vi "Finish.vi"(4 "error in (no error)":errorcluster) -> (0 "error out":errorcluster)   [LabVIEW 2016]
doc: "This VI is called just before exiting. It is expected to close I/O refnum, save collected data, etc."
uses:
  <vilib>/Rock Robotics/WPI/Utilities/WPI_GetSetVariantRefNum.vi
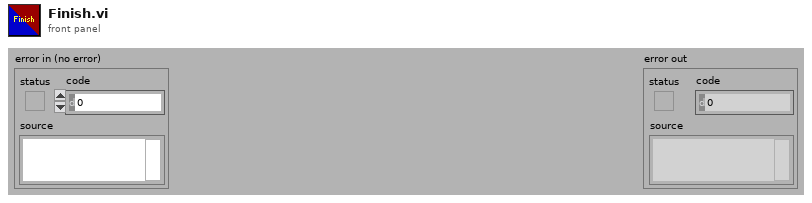
[diagram p1: front panel]
types:
  T1 = typedef "WPI_SolenoidDevRef.ctl" = cluster{"DevStatus":errorcluster, "Pneumatics Control Module":u8, "Forward Solenoid Channel":T2, "Reverse Solenoid Channel":T2}
  T2 = typedef "WPI_SolenoidChannel.ctl" = enum8{"Solenoid 0", "Solenoid 1", "Solenoid 2", "Solenoid 3", "Solenoid 4", "Solenoid 5", "Solenoid 6", "Solenoid 7", "Invalid"}
  T3 = typedef "WPI_JoystickDevRef.ctl" = cluster{"Device":T4}
  T4 = typedef "WPI_JoystickDeviceEnum.ctl" = enum16{"USB 0", "USB 1", "USB 2", "USB 3", "USB 4", "USB 5"}
  T5 = typedef "WPI_GyroDevRef.ctl" = cluster{"DevStatus":errorcluster, "Analog Channel":T6, "Offset":dbl, "Gain (VoltsPerDegree/Second)":dbl, "Gyro Type":enum16{"Analog", "XRS450"}, "Handle":i32, "SPI Bus":T7, "Device Found":bool, "Sample Rate":dbl, "Calibrate On Open":bool}
  T6 = typedef "FPGA_AIChannel.ctl" = enum8{"AI 0", "AI 1", "AI 2", "AI 3", "AI MXP 0", "AI MXP 1", "AI MXP 2", "AI MXP 3", "Invalid"}
  T7 = typedef "spi_bus.ctl" = enum16{"SPI On-Board, CS0", "SPI On-Board, CS1", "SPI On-Board, CS2", "SPI On-Board, CS3", "SPI MXP", "Invalid"}
  T8 = typedef "WPI_AccelerometerDevRef.ctl" = cluster{"DevStatus":errorcluster, "Scaling":T9, "Analog Channels":T10, "I2C Bus":T11, "SPI Bus":T7, "Accel Range":T12, "ADXL Axes":T13, "Handle":i32, "Device Address":u8, "Accel Type":enum16{"Analog", "ADXL345 I2C", "ADXL345 SPI", "Internal", "ADXL362 SPI"}}
  T9 = typedef "WPI_AccelerometerScaling.ctl" = cluster{"Gain (VoltsPerG)":dbl, "Center Voltage":dbl}
  T10 = typedef "WPI_AccelerometerAnalogChannels.ctl" = cluster{"X-Axis":T6, "Y-Axis":T6, "Z-Axis":T6}
  T11 = typedef "i2c_bus.ctl" = enum16{"I2C On-Board", "I2C MXP", "Invalid"}
  T12 = typedef "ADXL345 Range.ctl" = u8
  T13 = typedef "WPI_AccelerometerADXL345 Axes.ctl" = cluster{"X-Axis":bool, "Y-Axis":bool, "Z-Axis":bool}
  T14 = typedef "WPI_MotorControlDeviceRef.ctl" = cluster{"DeviceStatus":errorcluster, "Type":T15, "PWM":cluster{"PWM Channel":T16, "DeadBand":T17}, "CAN":cluster{"Device Number":u8, "SetOutput VI Ref":variant, "GetOutput VI Ref":variant, "Enable VI Ref":variant, "Disable VI Ref":variant, "Data":variant}, "Invert":bool}
  T15 = typedef "WPI_MotorControlType.ctl" = enum16{"PWM", "CAN"}
  T16 = typedef "FPGA_DIOPWMChannel.ctl" = enum8{"PWM 0", "PWM 1", "PWM 2", "PWM 3", "PWM 4", "PWM 5", "PWM 6", "PWM 7", "PWM 8", "PWM 9", "PWM MXP 0", "PWM MXP 1", "PWM MXP 2", "PWM MXP 3", "PWM MXP 4", "PWM MXP 5", "PWM MXP 6", "PWM MXP 7", "PWM MXP 8", "PWM MXP 9", "Invalid"}
  T17 = typedef "WPI_PWMDeadband.ctl" = cluster{"Name":string, "maxPositivePwm":i32, "minPositivePwm":i32, "centerPwm":i32, "maxNegativePwm":i32, "minNegativePwm":i32, "angularRange":u16}
  T18 = typedef "WPI_CompressorDevRef.ctl" = cluster{"DevStatus":errorcluster, "Pneumatics Control Module":u8}
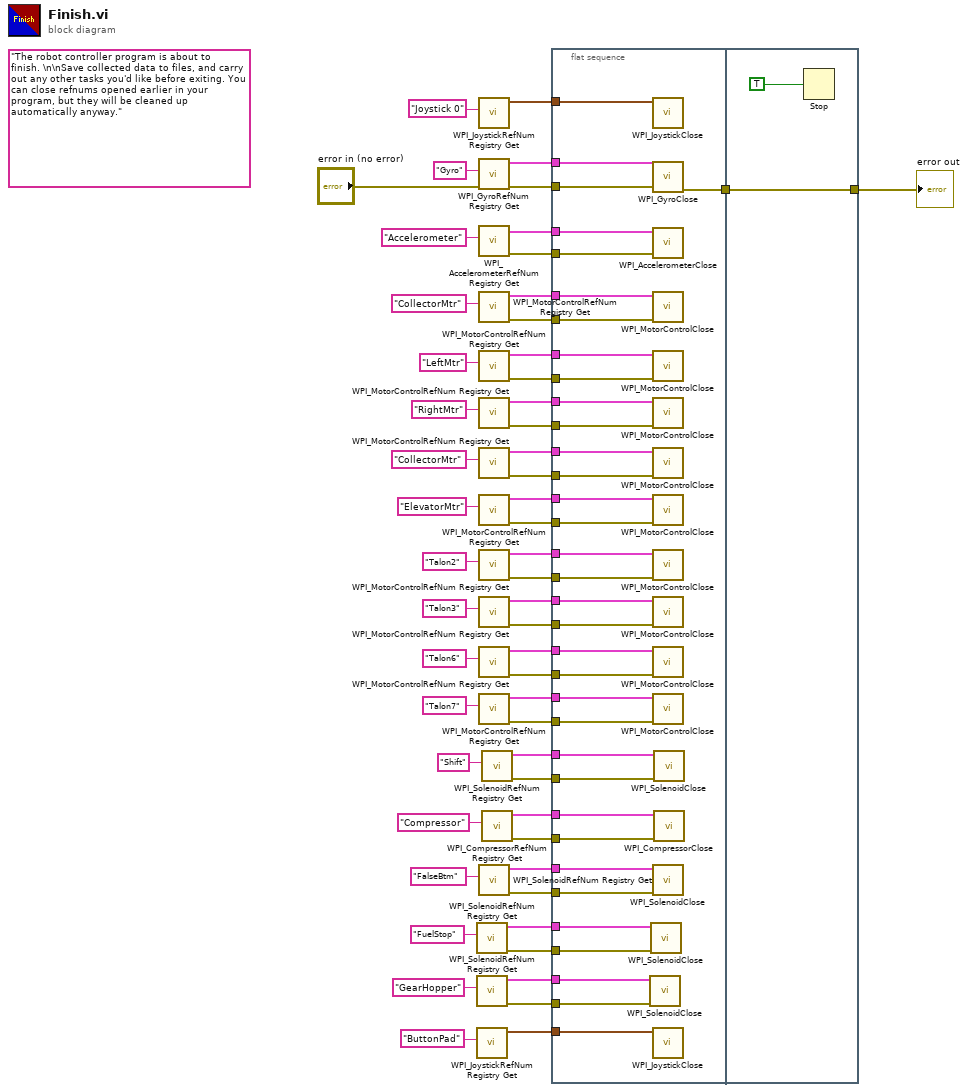
[diagram p0: block diagram]
diagram:
  (unwired) "The robot controller program is about to finish. \n\nSave collected data to files, and carry out any other tasks you'd like before exiting. You can close refnums opened earlier in your program, but they will be cleaned up automatically anyway."
  n1 = call <vilib>:"WPI_SolenoidRefNum Registry Get.vi"("refnum name"="FuelStop") -> ("error out"=w7:errorcluster, "SolenoidDevRef"=w8:T1)  [unwired: 9 in]
  n2 = call <vilib>:"WPI_SolenoidRefNum Registry Get.vi"("refnum name"="GearHopper") -> ("error out"=w9:errorcluster, "SolenoidDevRef"=w10:T1)  [unwired: 9 in]
  n3 = call <vilib>:"WPI_JoystickRefNum Registry Get.vi"("refnum name"="ButtonPad") -> ("JoystickDevRef"=w1:T3)  [unwired: 1 in, 9 out]
  n4 = call <vilib>:"WPI_JoystickRefNum Registry Get.vi"("refnum name"="Joystick 0") -> ("JoystickDevRef"=w54:T3)  [unwired: 1 in, 9 out]
  n5 = call <vilib>:"WPI_GyroRefNum Registry Get.vi"("error in (no error)"="error in (no error)", "refnum name"="Gyro") -> ("error out"=w3:errorcluster, "GyroDevRef"=w53:T5)  [unwired: 8 in]
  n6 = call <vilib>:"WPI_AccelerometerRefNum Registry Get.vi"("refnum name"="Accelerometer") -> ("error out"=w50:errorcluster, "AccelerometerDevRef"=w51:T8)  [unwired: 9 in]
  n7 = call <vilib>:"WPI_MotorControlRefNum Registry Get.vi"("refnum name"="CollectorMtr") -> ("error out"=w48:errorcluster, "MotorControlDevRef"=w47:T14)  [unwired: 9 in]
  n8 = call <vilib>:"WPI_MotorControlRefNum Registry Get.vi"("refnum name"="LeftMtr") -> ("error out"=w44:errorcluster, "MotorControlDevRef"=w43:T14)  [unwired: 9 in]
  n9 = call <vilib>:"WPI_MotorControlRefNum Registry Get.vi"("refnum name"="RightMtr") -> ("error out"=w41:errorcluster, "MotorControlDevRef"=w42:T14)  [unwired: 9 in]
  n10 = call <vilib>:"WPI_MotorControlRefNum Registry Get.vi"("refnum name"="CollectorMtr") -> ("error out"=w35:errorcluster, "MotorControlDevRef"=w36:T14)  [unwired: 9 in]
  n11 = call <vilib>:"WPI_MotorControlRefNum Registry Get.vi"("refnum name"="ElevatorMtr") -> ("error out"=w38:errorcluster, "MotorControlDevRef"=w37:T14)  [unwired: 9 in]
  n12 = call <vilib>:"WPI_MotorControlRefNum Registry Get.vi"("refnum name"="Talon2") -> ("error out"=w26:errorcluster, "MotorControlDevRef"=w27:T14)  [unwired: 9 in]
  n13 = call <vilib>:"WPI_MotorControlRefNum Registry Get.vi"("refnum name"="Talon3") -> ("error out"=w29:errorcluster, "MotorControlDevRef"=w28:T14)  [unwired: 9 in]
  n14 = call <vilib>:"WPI_MotorControlRefNum Registry Get.vi"("refnum name"="Talon6") -> ("error out"=w33:errorcluster, "MotorControlDevRef"=w32:T14)  [unwired: 9 in]
  n15 = call <vilib>:"WPI_MotorControlRefNum Registry Get.vi"("refnum name"="Talon7") -> ("error out"=w30:errorcluster, "MotorControlDevRef"=w31:T14)  [unwired: 9 in]
  n16 = call <vilib>:"WPI_SolenoidRefNum Registry Get.vi"("refnum name"="FalseBtm") -> ("error out"=w20:errorcluster, "SolenoidDevRef"=w21:T1)  [unwired: 9 in]
  n17 = call <vilib>:"WPI_SolenoidRefNum Registry Get.vi"("refnum name"="Shift") -> ("error out"=w15:errorcluster, "SolenoidDevRef"=w16:T1)  [unwired: 9 in]
  n18 = call <vilib>:"WPI_CompressorRefNum Registry Get.vi"("refnum name"="Compressor") -> ("error out"=w13:errorcluster, "CompressorDevRef"=w14:T18)  [unwired: 9 in]
  n19 = flat-sequence {
    tunnel: w54 -> [w90]
    tunnel: w53 -> [w89]
    tunnel: w51 -> [w88]
    tunnel: w50 -> [w87]
    tunnel: w48 -> [w86]
    tunnel: w47 -> [w85]
    tunnel: w44 -> [w84]
    tunnel: w43 -> [w83]
    tunnel: w41 -> [w81]
    tunnel: w42 -> [w82]
    tunnel: w35 -> [w77]
    tunnel: w36 -> [w78]
    tunnel: w38 -> [w80]
    tunnel: w37 -> [w79]
    tunnel: w26 -> [w69]
    tunnel: w27 -> [w70]
    tunnel: w29 -> [w72]
    tunnel: w28 -> [w71]
    tunnel: w33 -> [w76]
    tunnel: w32 -> [w75]
    tunnel: w30 -> [w73]
    tunnel: w31 -> [w74]
    tunnel: w20 -> [w67]
    tunnel: w21 -> [w68]
    tunnel: w16 -> [w66]
    tunnel: w15 -> [w65]
    tunnel: w14 -> [w64]
    tunnel: w13 -> [w63]
    tunnel: w10 -> [w62]
    tunnel: w9 -> [w61]
    tunnel: w8 -> [w60]
    tunnel: w7 -> [w59]
    tunnel: [w58] -> w4
    tunnel: w3 -> [w57]
    tunnel: w1 -> [w56]
    tunnel: [w91] -> w5
    tunnel: w4 -> [w91]
    frame #0 {
      n20 = call <vilib>:"WPI_SolenoidClose.vi"("error in (no error)"=w61, "SolenoidDevRef"=w62) -> ()  [unwired: 9 in, 1 out]
      n21 = call <vilib>:"WPI_SolenoidClose.vi"("error in (no error)"=w59, "SolenoidDevRef"=w60) -> ()  [unwired: 9 in, 1 out]
      n22 = call <vilib>:"WPI_JoystickClose.vi"("JoystickDevRef"=w90) -> ()  [unwired: 11 out]
      n23 = call <vilib>:"WPI_GyroClose.vi"("error in"=w57, "GyroDevRef"=w89) -> ("error out"=w58:errorcluster)  [unwired: 9 in]
      n24 = call <vilib>:"WPI_AccelerometerClose.vi"("error in"=w87, "AccelerometerDevRef"=w88) -> ()  [unwired: 9 in, 1 out]
      n25 = call <vilib>:"WPI_MotorControlClose.vi"("error in"=w86, "MotorControlDevRef"=w85) -> ()  [unwired: 9 in, 1 out]
      n26 = call <vilib>:"WPI_MotorControlClose.vi"("error in"=w84, "MotorControlDevRef"=w83) -> ()  [unwired: 9 in, 1 out]
      n27 = call <vilib>:"WPI_MotorControlClose.vi"("error in"=w81, "MotorControlDevRef"=w82) -> ()  [unwired: 9 in, 1 out]
      n28 = call <vilib>:"WPI_MotorControlClose.vi"("error in"=w77, "MotorControlDevRef"=w78) -> ()  [unwired: 9 in, 1 out]
      n29 = call <vilib>:"WPI_MotorControlClose.vi"("error in"=w80, "MotorControlDevRef"=w79) -> ()  [unwired: 9 in, 1 out]
      n30 = call <vilib>:"WPI_MotorControlClose.vi"("error in"=w69, "MotorControlDevRef"=w70) -> ()  [unwired: 9 in, 1 out]
      n31 = call <vilib>:"WPI_MotorControlClose.vi"("error in"=w72, "MotorControlDevRef"=w71) -> ()  [unwired: 9 in, 1 out]
      n32 = call <vilib>:"WPI_MotorControlClose.vi"("error in"=w76, "MotorControlDevRef"=w75) -> ()  [unwired: 9 in, 1 out]
      n33 = call <vilib>:"WPI_MotorControlClose.vi"("error in"=w73, "MotorControlDevRef"=w74) -> ()  [unwired: 9 in, 1 out]
      n34 = call <vilib>:"WPI_SolenoidClose.vi"("error in (no error)"=w67, "SolenoidDevRef"=w68) -> ()  [unwired: 9 in, 1 out]
      n35 = call <vilib>:"WPI_JoystickClose.vi"("JoystickDevRef"=w56) -> ()  [unwired: 11 out]
      n36 = call <vilib>:"WPI_SolenoidClose.vi"("error in (no error)"=w65, "SolenoidDevRef"=w66) -> ()  [unwired: 9 in, 1 out]
      n37 = call <vilib>:"WPI_CompressorClose.vi"("error in (no error)"=w63, "CompressorDevRef"=w64) -> ()  [unwired: 9 in, 1 out]
    }
    frame #1 {
      n38 = Stop(stop? (T)=TRUE ("Quit")) -> ()
    }
  }
  "error out" <- w5
